vi "Legend.vi"(0 "reference in":refnum<class "HTMLPlot.lvclass">, 1 "Position":T1=enum."bottom", 5 "error in (no error)":errorcluster, 6 "Show(T)":bool=TRUE) -> (14 "reference out":refnum<class "HTMLPlot.lvclass">, 19 "error out":errorcluster)   [LabVIEW 2019, in "HTMLPlot.lvclass"]
uses:
  HTMLPlot.lvclass
  Controls/LegendPosition.ctl
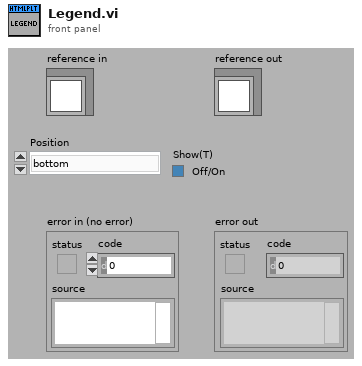
[diagram p1: front panel]
types:
  T1 = typedef "HTMLPlot.lvclass/LegendPosition.ctl" = enum16{"top", "right", "left", "bottom"}
  T2 = typedef "HTMLPlot.lvclass/ObjectAttributes.ctl" = cluster{"Attribute1":dbl, "GraphContainer":refnum<k7>, "ChartScriptFile":string, "UtilScriptFile(demoData)":string, "BaseHTML":string, "GenericProperties":cluster{"PlotType":T3, "PlotTitle":string, "XLabel":string, "YLabel":string, "ShowToolTip":bool}, "LegendProperties":cluster{"Show":bool, "Position":T1}, "BarPlot":cluster{"Dataset":dbl[][], "DatasetLabels":string[], "XLabels":string[], "PlotColours":u32[], "Stacked":bool}, "PiePlot":cluster{"Dataset":dbl[][], "DatasetLabels":string[], "PlotColours":u32[], "DoughnutStyle":bool, "PlotLabels":string[]}, "connection ID":refnum<k5>, "PortID":u64}
  T3 = typedef "HTMLPlot.lvclass/PlotType.ctl" = enum16{"bar", "line", "pie"}
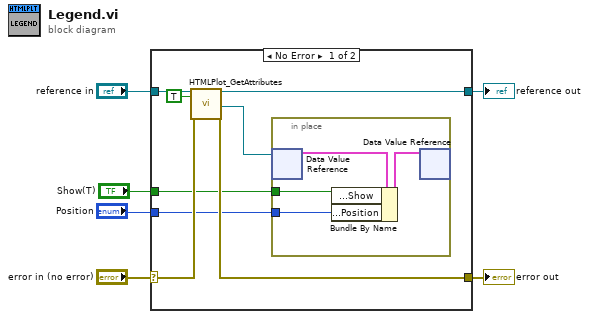
[diagram p0: block diagram]
diagram:
  n1 = case shown="No Error" "error in (no error)" {
    selector: "error in (no error)" -> [w14 w20]
    tunnel: [w13 w20] -> w5
    tunnel: [w11 w19] -> w3
    tunnel: "reference in" -> [w12 w19]
    tunnel: "Show(T)" -> [w8 _]
    tunnel: "Position" -> [w7 _]
    frame No Error {
      n2 = call "HTMLPlot_GetAttributes.vi"("reference in"=w12, "OnlyGetDvrReference(False)"=TRUE, "error in (no error)"=w14) -> ("reference out"=w11:refnum<class "HTMLPlot.lvclass">, "DataRef"=w10:refnum<data-value>, "error out"=w13:errorcluster)  [unwired: 13 in, 1 out]
      n3 = in-place {
        in-place-border: w8 -> [w16]
        in-place-border: w7 -> [w15]
        n4 = in-place-dvr #1(w10) -> (w18:T2)  [unwired: 1 out]
        n5 = Bundle By Name(cluster=w18, "LegendProperties.Show"=w16, "LegendProperties.Position"=w15) -> (w17:T2)
        n6 = in-place-dvr #1(w17) -> ()  [unwired: 2 out]
      }
    }
    frame Error {
    }
  }
  "error out" <- w5
  "reference out" <- w3
